vi "TWM Client Cmd Set Corrections.vi"(4 "set digitizer (True)":bool=TRUE, 5 "timeout [ms]":i32=5000, 6 "set transducers (True)":bool, 7 "end of packet key":string="TWM:command:EndOfPacket", 8 "error in":errorcluster, 9 "digitizer correction":path, 10 "list of transducers":T1[](array[typedef]), 11 "handle":i32) -> (0 "error out":errorcluster, 3 "handle out":i32)   [LabVIEW 2020, in "TWM Client.lvlib"]
doc: "Write Set corrections command packet to TWM server. Wait for ACK. \"Set*\" flags must be set to actually send the command. Note the virtual channel indices in the transducer list are optional. Zero value means the low-side is disabled (single-ended mode). Zero value for high-side means the order of virtual channels will be generated automatically."
uses:
  TWM Client.lvlib
  TWM Client Transducer Correction Item.ctl
  octave/infolib/1D I64.vi
  octave/infolib/1D String.vi
  octave/infolib/String.vi
  octave/infolib/infolib.lvlib
panel:
  out "info data out":string
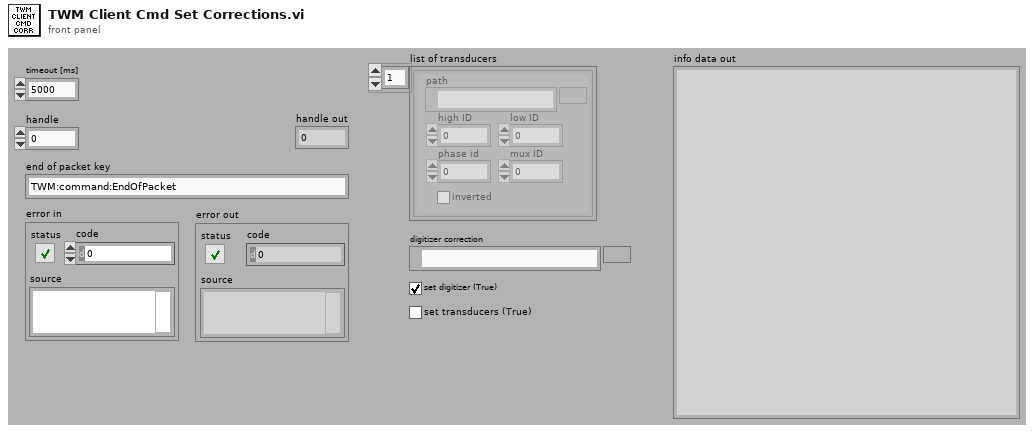
[diagram p1: front panel]
types:
  T1 = typedef "TWM Client.lvlib/TWM Client Transducer Correction Item.ctl" = cluster{"path":path, "high ID":i32, "low ID":i32, "phase id":i32, "mux ID":i32, "inverted":bool}
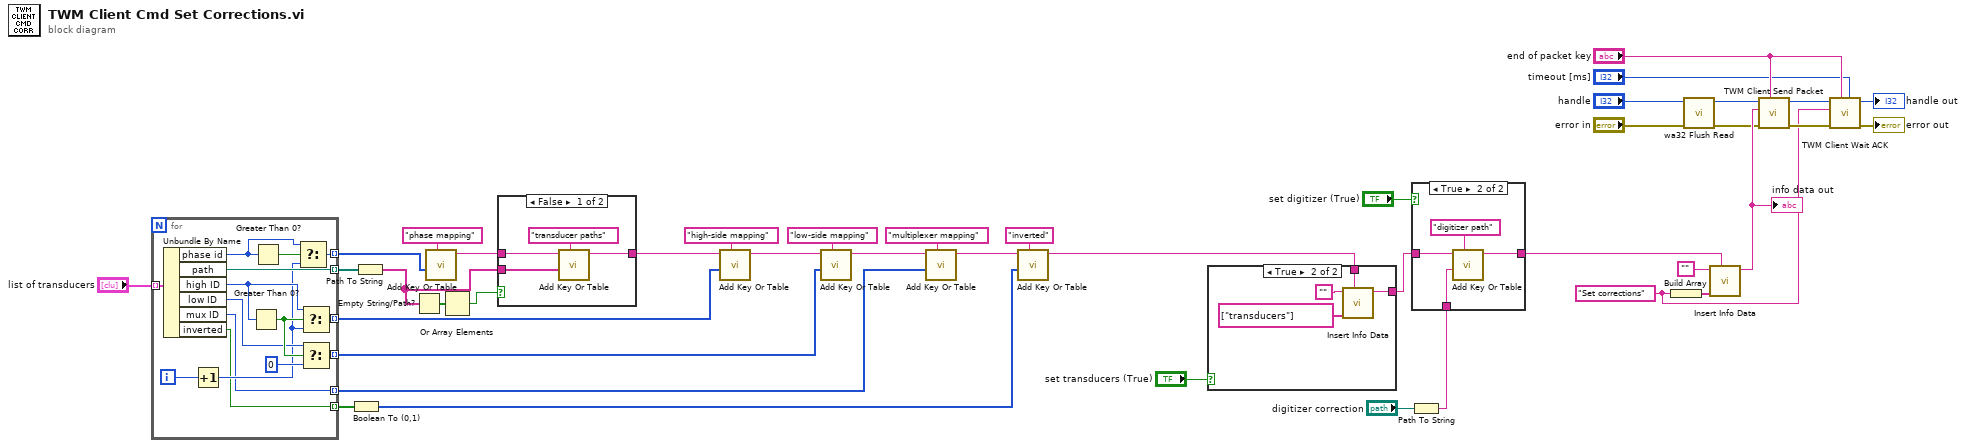
[diagram p0: block diagram]
diagram:
  w22 = "Set corrections" ("section name")
  n1 = for {
    tunnel: "list of transducers" -> [w57] mode=indexing
    tunnel: [w51] -> w14 mode=indexing
    tunnel: [w50] -> w40 mode=indexing
    tunnel: [w49] -> w37 mode=indexing
    tunnel: [w45] -> w17 mode=indexing
    tunnel: [w44] -> w15 mode=indexing
    tunnel: [w43] -> w2 mode=indexing
    i -> [w55]
    n2 = Unbundle By Name(w57) -> ("phase id"=w47:i32, "path"=w51:path, "high ID"=w56:i32, "low ID"=w53:i32, "mux ID"=w44:i32, "inverted"=w43:bool)
    n3 = Increment(x=w55) -> (x+1=w46:i32)
    n4 = Greater Than 0?(x=w56) -> (x > 0?=w54:bool)
    n5 = Greater Than 0?(x=w47) -> (x > 0?=w48:bool)
    n6 = Select(t=w47, s=w48, f=w46) -> (s? t:f=w45:i32)
    n7 = Select(t=w56, s=w54, f=w46) -> (s? t:f=w50:i32)
    n8 = Select(t=w53, s=w54, f=0) -> (s? t:f=w49:i32)
  }
  n9 = Boolean To (0,1)(Boolean=w2) -> (0, 1=w1:i16[])
  n10 = Path To String(path=w14) -> (string=w13:string[])
  n11 = Empty String/Path?(string/path=w13) -> (empty?=w12:bool[])
  n12 = call-poly "Add Key Or Table.vi"("key description"="phase mapping", "numeric"=w17) -> ("info data out"=w18:string)  [unwired: 8 in, 1 out]
  n13 = Or Array Elements(Boolean array=w12) -> (logical OR=w11:bool)
  n14 = case shown="False" w11 {
    tunnel: [w60 w62] -> w41
    tunnel: w18 -> [w59 w62]
    tunnel: w13 -> [w58 _]
    frame False {
      n15 = call-poly "Add Key Or Table.vi"("key description"="transducer paths", "string"=w58, "info data"=w59) -> ("info data out"=w60:string)  [unwired: 7 in, 1 out]
    }
    frame True {
    }
  }
  n16 = call-poly "Add Key Or Table.vi"("key description"="high-side mapping", "numeric"=w40, "info data"=w41) -> ("info data out"=w36:string)  [unwired: 7 in, 1 out]
  n17 = call-poly "Add Key Or Table.vi"("key description"="low-side mapping", "numeric"=w37, "info data"=w36) -> ("info data out"=w16:string)  [unwired: 7 in, 1 out]
  n18 = call-poly "Add Key Or Table.vi"("key description"="multiplexer mapping", "numeric"=w15, "info data"=w16) -> ("info data out"=w4:string)  [unwired: 7 in, 1 out]
  n19 = call-poly "Add Key Or Table.vi"("key description"="inverted", "numeric"=w1, "info data"=w4) -> ("info data out"=w3:string)  [unwired: 7 in, 1 out]
  n20 = case shown="True" "set transducers (True)" {
    tunnel: w3 -> [_ w66]
    tunnel: [_ w64] -> w34
    frame False {
    }
    frame True {
      n21 = call "Insert Info Data.vi"("info data to insert"=w66, "sections"=string[] ["transducers"], "info data"="") -> ("info data out"=w64:string)  [unwired: 7 in, 1 out]
    }
  }
  n22 = Path To String(path="digitizer correction") -> (string=w31:string)
  n23 = case shown="True" "set digitizer (True)" {
    tunnel: w34 -> [w67 w71]
    tunnel: [w67 w69] -> w30
    tunnel: w31 -> [_ w68]
    frame False {
    }
    frame True {
      n24 = call-poly "Add Key Or Table.vi"("key description"="digitizer path", "string"=w68, "info data"=w71) -> ("info data out"=w69:string)  [unwired: 7 in, 1 out]
    }
  }
  n25 = Build Array(w22) -> (w28:string[])
  n26 = call "wa32 Flush Read.vi"("error in"="error in", "handle"="handle") -> ("error out"=w8:errorcluster, "handle out"=w7:i32)  [unwired: 7 in, 1 out]
  n27 = call "Insert Info Data.vi"("info data to insert"=w30, "sections"=w28, "info data"="") -> ("info data out"=w29:string)  [unwired: 7 in, 1 out]
  "info data out" <- w29
  n28 = call "TWM Client Send Packet.vi"("end of packet key"="end of packet key", "error in"=w8, "command string"=w29, "handle"=w7) -> ("error out"=w24:errorcluster, "handle out"=w21:i32)  [unwired: 6 in]
  n29 = call "TWM Client Wait ACK.vi"("timeout [ms] (3000)"="timeout [ms]", "key string"="end of packet key", "error in"=w24, "command header"=w22, "handle"=w21) -> ("error out"=→"error out":errorcluster, "handle out"=→"handle out":i32)  [unwired: 5 in]
